vi "Begin.vi"(11 "Image Size":T1=enum."160x120") -> (0 "error out":errorcluster)   [LabVIEW 2012]
doc: "Called before other user functions, this VI is expected to open initial I/O refnums, load in file data, and do all program initialization. Notice that the <B>error out</B> terminal is simply used for data flow. Wiring it to other structures or subVIs ensures that this VI runs first."
uses:
  <vilib>/Rock Robotics/WPI/Camera/WPI_CameraImageSize.ctl
  <vilib>/Rock Robotics/WPI/Camera/WPI_CameraWhite Balance Values.ctl
  <vilib>/Rock Robotics/WPI/Camera/WPI_CameraExposure Values.ctl
  <vilib>/Rock Robotics/WPI/Camera/WPI_CameraFrameRate.ctl
  <vilib>/Rock Robotics/WPI/DriverStation/WPI_DriverStationRobotMode2.ctl
  <vilib>/Rock Robotics/WPI/Joystick/WPI_JoystickDeviceEnum.ctl
  <vilib>/Rock Robotics/SystemInterfaces/DIO/FPGA_DIOPWMChannel.ctl
  <vilib>/Rock Robotics/WPI/Solenoid/WPI_SolenoidChannel.ctl
  <vilib>/Rock Robotics/SystemInterfaces/DIO/FPGA_DIORelayChannel.ctl
  <vilib>/Rock Robotics/WPI/Relay/WPI_RelayDirection.ctl
  <vilib>/Rock Robotics/SystemInterfaces/DIO/FPGA_DIOChannel.ctl
  <vilib>/Rock Robotics/WPI/Encoder/WPI_EncoderType.ctl
  <vilib>/Rock Robotics/SystemInterfaces/Typedef/FPGA_TypedefDigitalModule.ctl
  <vilib>/Rock Robotics/SystemInterfaces/Typedef/FPGA_TypedefAnalogModuleForGyro.ctl
  <vilib>/Rock Robotics/SystemInterfaces/AI/FPGA_AIGyroChannel.ctl
  <vilib>/Rock Robotics/SystemInterfaces/Typedef/FPGA_TypedefSolenoidModule.ctl
  Robot Global Data.vi
  <vilib>/Rock Robotics/WPI/RobotDrive/WPI_RobotDriveOpen4MotorWithTalon.vi
  <vilib>/Rock Robotics/WPI/MotorControl/WPI_MotorControlOpen Talon.vi
  <vilib>/Rock Robotics/WPI/Solenoid/WPI_SolenoidOpenSingle.vi
  <vilib>/Rock Robotics/WPI/Solenoid/Deprecated/WPI_SolenoidSetBool.vi
  <vilib>/Rock Robotics/WPI/Counter/WPI_CounterDigitalInputToDigitalSource.vi
  <vilib>/Rock Robotics/WPI/MotorControl/WPI_MotorControlOpen Jaguar.vi
  <vilib>/Rock Robotics/WPI/Compressor/WPI_CompressorGetSetRefNum.vi
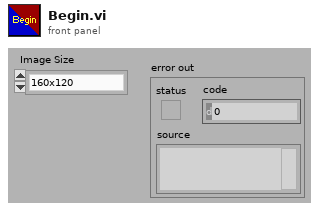
[diagram p1: front panel]
types:
  T1 = typedef "WPI_CameraImageSize.ctl" = enum16{"640x480", "320x240", "160x120"}
  T2 = typedef "FPGA_TypedefSolenoidModule.ctl" = enum16{"Solenoid Module 1", "Solenoid Module 2"}
  T3 = typedef "WPI_SolenoidChannel.ctl" = enum8{"Solenoid 1", "Solenoid 2", "Solenoid 3", "Solenoid 4", "Solenoid 5", "Solenoid 6", "Solenoid 7", "Solenoid 8", "Invalid"}
  T4 = typedef "FPGA_DIOPWMChannel.ctl" = enum8{"PWM 1", "PWM 2", "PWM 3", "PWM 4", "PWM 5", "PWM 6", "PWM 7", "PWM 8", "PWM 9", "PWM 10", "Invalid"}
  T5 = typedef "FPGA_TypedefDigitalModule.ctl" = enum16{"Digital Module 1", "Digital Module 2"}
  T6 = typedef "FPGA_AIGyroChannel.ctl" = enum8{"AI 1", "AI 2", "Invalid"}
  T7 = typedef "FPGA_TypedefAnalogModuleForGyro.ctl" = enum16{"Analog Module 1"}
  T8 = typedef "WPI_EncoderType.ctl" = enum16{"1x", "2x", "4x"}
  T9 = typedef "FPGA_DIOChannel.ctl" = enum8{"DIO 1", "DIO 2", "DIO 3", "DIO 4", "DIO 5", "DIO 6", "DIO 7", "DIO 8", "DIO 9", "DIO 10", "DIO 11", "DIO 12", "DIO 13", "DIO 14", "Invalid"}
  T10 = typedef "FPGA_DIORelayChannel.ctl" = enum8{"Relay 1", "Relay 2", "Relay 3", "Relay 4", "Relay 5", "Relay 6", "Relay 7", "Relay 8", "Invalid"}
  T11 = typedef "WPI_JoystickDeviceEnum.ctl" = enum16{"USB 1", "USB 2", "USB 3", "USB 4", "Kinect 1", "Kinect 2"}
  T12 = typedef "WPI_RelayDirection.ctl" = enum16{"Both directions", "Forward only", "Reverse only"}
  T13 = typedef "WPI_DriverStationRobotMode2.ctl" = enum16{"Autonomous Disabled", "Autonomous Enabled", "Teleop Disabled", "Teleop Enabled", "Timeout", "Finish", "Test Disabled", "Test Enabled"}
  T14 = typedef "WPI_CameraFrameRate.ctl" = u32
  T15 = typedef "WPI_CameraExposure Values.ctl" = enum16{"Auto", "Flicker-free 50 Hz", "Flicker-free 60 Hz", "Hold current"}
  T16 = typedef "WPI_CameraWhite Balance Values.ctl" = enum16{"Auto", "Fixed indoor", "Fixed outdoor 1", "Fixed outdoor 2", "Fixed fluorescent 1", "Fixed fluorescent 2", "Hold current"}
  T17 = typedef "WPI_MotorControlDeviceRef.ctl" = cluster{"DeviceStatus":errorcluster, "Type":enum16{"PWM", "CAN"}, "PWM":cluster{"Digital Module":T5, "PWM Channel":T4, "DeadBand":T18}, "CAN":cluster{"Device Number":u8, "Control Mode":T19, "Semaphore":T20, "Max Vout":dbl}, "Invert":bool, "TransformRef":T21, "InvTransformRef":T21}
  T18 = typedef "WPI_PWMDeadband.ctl" = cluster{"Name":string, "maxPositivePwm":i32, "minPositivePwm":i32, "centerPwm":i32, "maxNegativePwm":i32, "minNegativePwm":i32, "angularRange":u16}
  T19 = typedef "WPI_CANJaguar_ControlMode.ctl" = enum8{"Percent VBus", "Current", "Speed", "Position", "Voltage"}
  T20 = typedef "Semaphore RefNum" = refnum<k1>
  T21 = typedef "WPI_PWMTransform_ConPane.ctl" = refnum<vi>
  T22 = typedef "WPI_DigitalInputDevRef.ctl" = cluster{"DevStatus":errorcluster, "DIO Channel":T9, "Digital Module":T5}
  T23 = typedef "WPI_ServoDeviceRef.ctl" = cluster{"DeviceStatus":errorcluster, "Digital Module":T5, "PWM Channel":T4, "DeadBand":T18}
  T24 = typedef "WPI_JoystickDevRef.ctl" = cluster{"Device":T11}
  T25 = typedef "WPI_GyroDevRef.ctl" = cluster{"DevStatus":errorcluster, "Analog Module":T26, "Analog Channel":T27, "Offset":dbl, "Gain (VoltsPerDegree/Second)":dbl}
  T26 = typedef "FPGA_TypedefAnalogModule.ctl" = enum16{"Analog Module 1", "Analog Module 2"}
  T27 = typedef "FPGA_AIChannel.ctl" = enum8{"AI 1", "AI 2", "AI 3", "AI 4", "AI 5", "AI 6", "AI 7", "AI 8", "Invalid"}
  T28 = typedef "FPGA_CounterEncoderSourceConvertionLVSourceType.ctl" = cluster{"DevStatus":errorcluster, "AnalogTriggerMode?":bool, "DigitalMode":cluster{"Digital Module":T5, "DIO Channel":T29}, "AnalogTriggerMode":cluster{"AnalogTriggerIndex":T30, "OutputType":T31}}
  T29 = typedef "FPGA_DIODigitalSourceChannel.ctl" = enum8{"DIO 1", "DIO 2", "DIO 3", "DIO 4", "DIO 5", "DIO 6", "DIO 7", "DIO 8", "DIO 9", "DIO 10", "DIO 11", "DIO 12", "DIO 13", "DIO 14", "Disabled"}
  T30 = typedef "FPGA_AnalogTriggerIndex.ctl" = enum8{"Trig 0", "Trig 1", "Trig 2", "Trig 3", "Trig 4", "Trig 5", "Trig 6", "Trig 7", "Invalid"}
  T31 = typedef "FPGA_AnalogTriggerOutType.ctl" = enum16{"InWindow", "TriggerState", "Rising", "Falling"}
  T32 = typedef "WPI_SolenoidDevRef.ctl" = cluster{"DevStatus":errorcluster, "Solenoid Module":T2, "Forward Solenoid Channel":T3, "Reverse Solenoid Channel":T3}
  T33 = typedef "WPI_CompressorDevRef.ctl" = cluster{"DevStatus":errorcluster, "DigitalInputDevRef":T22, "RelayDevRef":T34}
  T34 = typedef "WPI_RelayDevRef.ctl" = cluster{"DevStatus":errorcluster, "Relay Channel":T10, "Digital Module":T5, "Relay Direction":T12}
  T35 = typedef "WPI_RobotDriveDevRef.ctl" = cluster{"DevStatus":errorcluster, "Motors[]":T17[], "Square Inputs":bool, "Max Output":dbl, "Isochronous":bool}
  T36 = typedef "WPI_EncoderDevRef.ctl" = cluster{"DevStatus":errorcluster, "EncoderIndex":T37, "CounterIndex":T38, "DistancePerCount":dbl, "Decoding Type":T8}
  T37 = typedef "FPGA_EncoderIdx.ctl" = enum8{"Enc 0", "Enc 1", "Enc 2", "Enc 3", "Invalid"}
  T38 = typedef "FPGA_CounterCtrSystemIndex.ctl" = enum8{"Ctr 0", "Ctr 1", "Ctr 2", "Ctr 3", "Ctr 4", "Ctr 5", "Ctr 6", "Ctr 7", "Invalid"}
  T39 = typedef "WPI_CameraDevRef.ctl" = cluster{"Camera Address":string, "CameraStatus":errorcluster, "Acquire Image Notifier":refnum<notifier>}
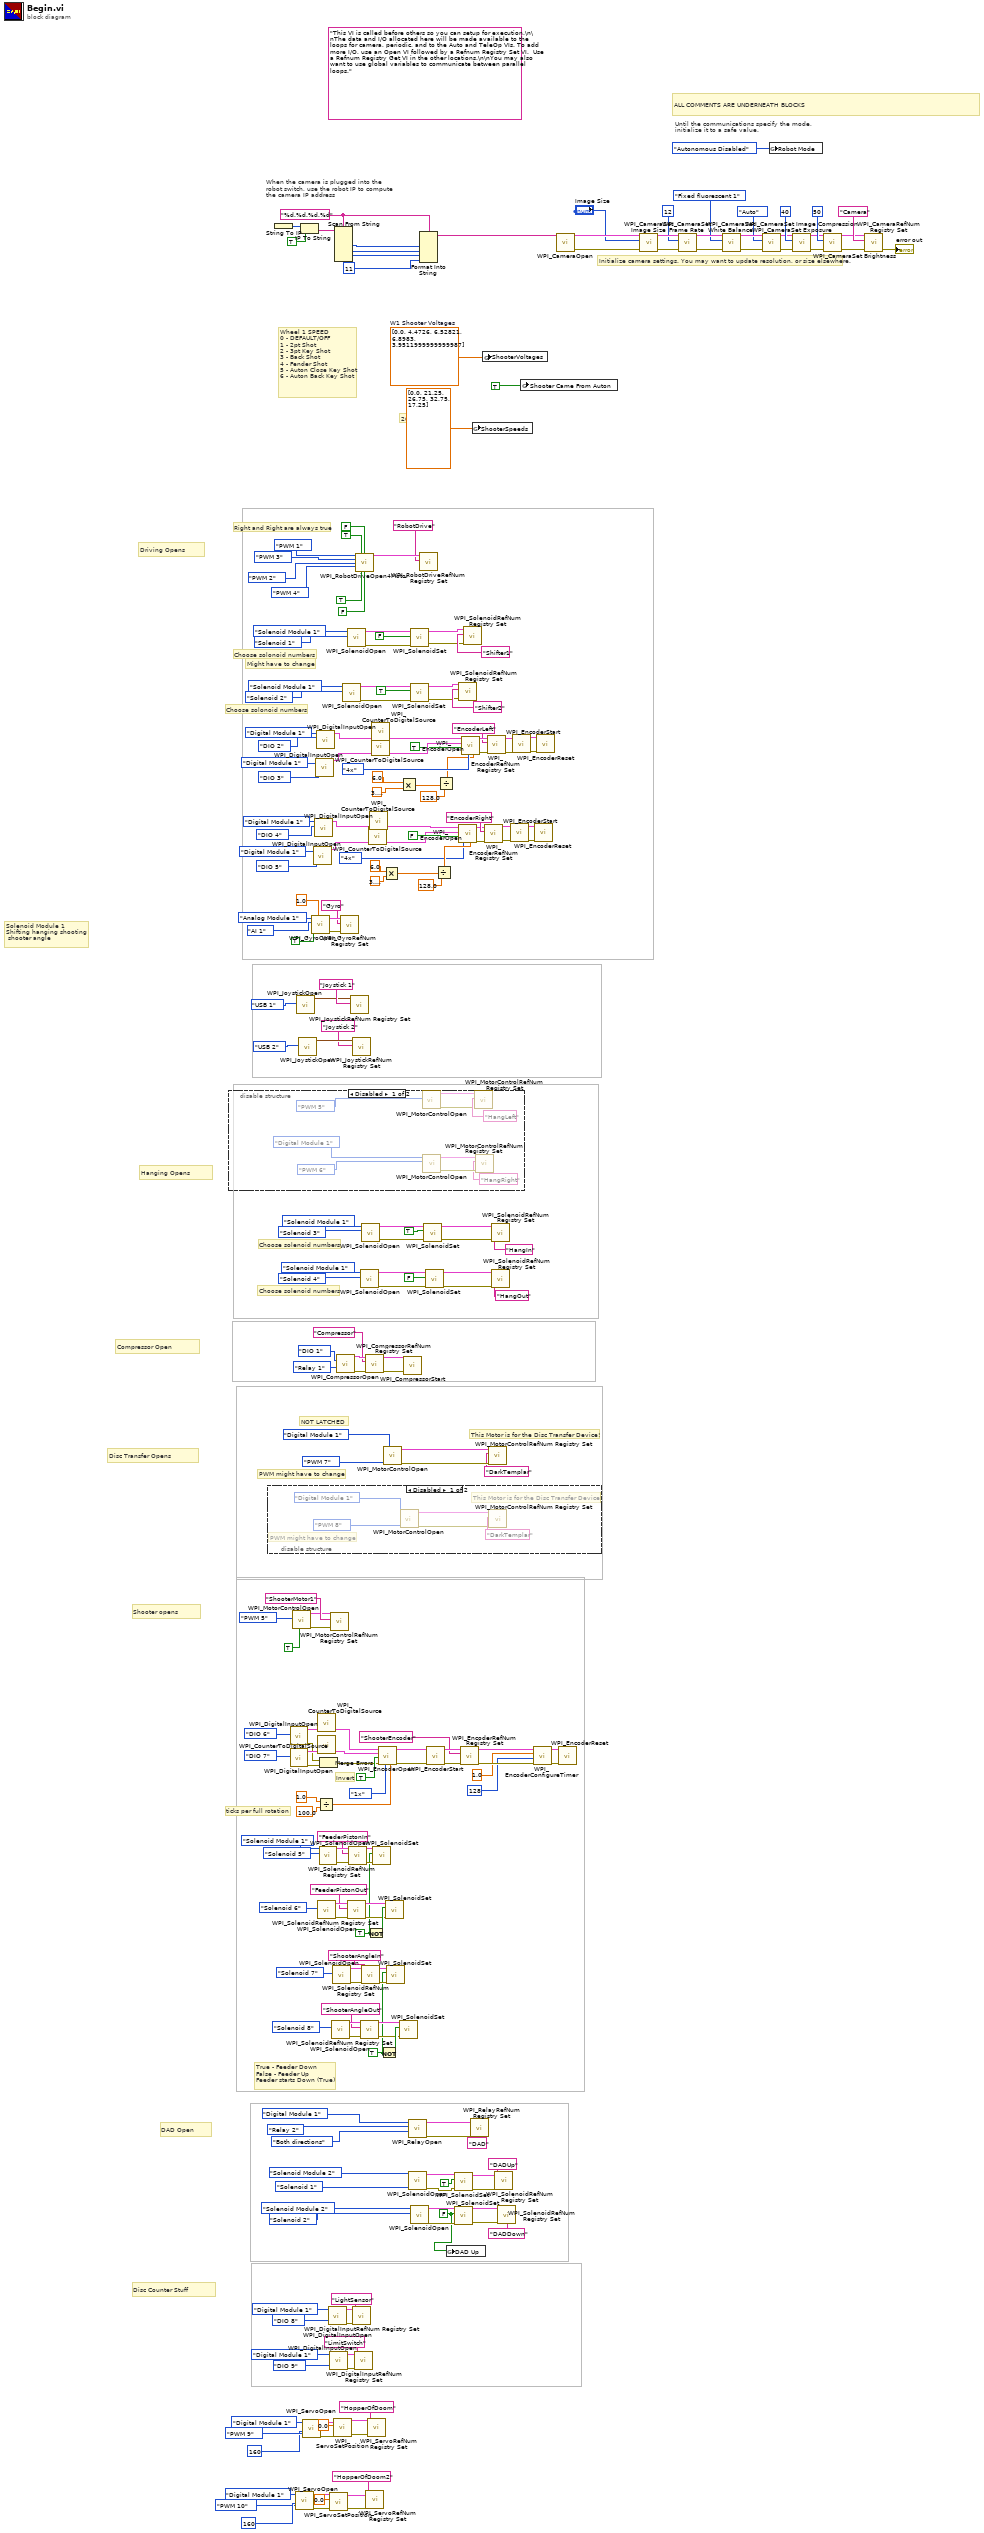
[diagram p0: block diagram]
diagram:
  w2 = TRUE
  w16 = TRUE
  w50 = FALSE
  w150 = dbl[] [0.0, 4.4726, 6.52821, 6.8983, 3.9511999999999987]  # W1 Shooter Voltages
  w227 = "%d.%d.%d.%d" ("format string")
  (unwired) "This VI is called before others so you can setup for execution.\n\nThe data and I/O allocated here will be made available to the loops for camera, periodic, and to the Auto and TeleOp VIs. To add more I/O, use an Open VI followed by a Refnum Registry Set VI.  Use a Refnum Registry Get VI in the other locations.\n\nYou may also want to use global variables to communicate between parallel loops."
  # "Solenoid Module 1\nShifting hanging shooting \n shooter angle"
  # "True - Feeder Down\nFalse - Feeder Up\nFeeder starts Down (True)"
  # "NOT LATCHED"
  # "Choose solenoid numbers"
  # "Choose solenoid numbers"
  # "Disc Counter Stuff"
  # "Compressor Open"
  # "26.75"
  # "Wheel 1 SPEED\n0 - DEFAULT/OFF\n1 - 2pt Shot\n2 - 3pt Key Shot\n3 - Back Shot\n4 - Fender Shot\n5 - Auton Close Key Shot\n6 - Auton Back Key Shot"
  # "Disc Transfer Opens"
  # "DAD Open"
  # "Hanging Opens"
  # "Driving Opens"
  # "Shooter opens"
  # "Invert"
  # "ticks per full rotation"
  # "Choose solonoid numbers"
  # "Might have to change"
  # "Choose solonoid numbers"
  # "PWM might have to change"
  # "ALL COMMENTS ARE UNDERNEATH BLOCKS"
  # "This Motor is for the Disc Transfer Device!"
  # "Right and Right are always true"
  # "Until the communications specify the mode,\ninitialize it to a safe value."
  # "When the camera is plugged into the\nrobot switch, use the robot IP to compute\nthe camera IP address"
  # "Initialize camera settings. You may want to update resolution, or size elsewhere."
  n1 = disable-structure shown="Disabled" {
    frame Disabled {
      n2 = call-poly <vilib>:"WPI_MotorControlOpen.vi"("PWM Channel"=FPGA_DIOPWMChannel."PWM 5") -> ("error out"=w258:errorcluster, "MotorControlDeviceRef"=w257:T17)  [unwired: 9 in]
      n3 = call-poly <vilib>:"WPI_MotorControlOpen.vi"("PWM Channel"=FPGA_DIOPWMChannel."PWM 6", "Digital Module (Module 1)"=FPGA_TypedefDigitalModule."Digital Module 1") -> ("error out"=w261:errorcluster, "MotorControlDeviceRef"=w262:T17)  [unwired: 8 in]
      n4 = call <vilib>:"WPI_MotorControlRefNum Registry Set.vi"("error in (no error)"=w258, "refnum name"="HangLeft", "MotorControlDevRef"=w257) -> ()  [unwired: 7 in, 2 out]
      n5 = call <vilib>:"WPI_MotorControlRefNum Registry Set.vi"("error in (no error)"=w261, "refnum name"="HangRight", "MotorControlDevRef"=w262) -> ()  [unwired: 7 in, 2 out]
    }
    frame Enabled {
    }
  }
  n6 = disable-structure shown="Disabled" {
    frame Disabled {
      # "PWM might have to change"
      # "This Motor is for the Disc Transfer Device!"
      n7 = call-poly <vilib>:"WPI_MotorControlOpen.vi"("PWM Channel"=FPGA_DIOPWMChannel."PWM 8", "Digital Module (Module 1)"=FPGA_TypedefDigitalModule."Digital Module 1") -> ("error out"=w268:errorcluster, "MotorControlDeviceRef"=w267:T17)  [unwired: 8 in]
      n8 = call <vilib>:"WPI_MotorControlRefNum Registry Set.vi"("error in (no error)"=w268, "refnum name"="DarkTemplar", "MotorControlDevRef"=w267) -> ()  [unwired: 7 in, 2 out]
    }
    frame Enabled {
    }
  }
  n9 = String To IP() -> (0:w234:u32)  [unwired: 1 in]
  n10 = call <vilib>:"WPI_DigitalInputOpen.vi"("DIO Channel"=FPGA_DIOChannel."DIO 6") -> ("error out"=w169:errorcluster, "DigitalInputDevRef"=w183:T22)  [unwired: 9 in]
  n11 = call <vilib>:"WPI_DigitalInputOpen.vi"("DIO Channel"=FPGA_DIOChannel."DIO 7") -> ("error out"=w168:errorcluster, "DigitalInputDevRef"=w179:T22)  [unwired: 9 in]
  n12 = call-poly <vilib>:"WPI_MotorControlOpen.vi"("Invert"=TRUE, "PWM Channel"=FPGA_DIOPWMChannel."PWM 5") -> ("error out"=w162:errorcluster, "MotorControlDeviceRef"=w163:T17)  [unwired: 8 in]
  n13 = call <vilib>:"WPI_ServoOpen.vi"("Angular Range"=160, "PWM Channel"=FPGA_DIOPWMChannel."PWM 10", "Digital Module (Module 1)"=FPGA_TypedefDigitalModule."Digital Module 1") -> ("error out"=w35:errorcluster, "ServoDeviceRef"=w34:T23)  [unwired: 7 in]
  n14 = call <vilib>:"WPI_JoystickOpen.vi"("JoystickDevice"=WPI_JoystickDeviceEnum."USB 1") -> ("JoystickDevRef"=w223:T24)  [unwired: 10 in]
  n15 = call <vilib>:"WPI_JoystickOpen.vi"("JoystickDevice"=WPI_JoystickDeviceEnum."USB 2") -> ("JoystickDevRef"=w152:T24)  [unwired: 10 in]
  n16 = IP To String(1:TRUE ("dot notation? (F)"), 2:w234) -> (0:w232:string)
  n17 = call <vilib>:"WPI_ServoOpen.vi"("Angular Range"=160, "PWM Channel"=FPGA_DIOPWMChannel."PWM 9", "Digital Module (Module 1)"=FPGA_TypedefDigitalModule."Digital Module 1") -> ("error out"=w39:errorcluster, "ServoDeviceRef"=w38:T23)  [unwired: 7 in]
  n18 = call <vilib>:"WPI_GyroOpen.vi"("Calibration Time (s)"=1.0, "Calibrate On Open"=TRUE, "Analog Channel"=FPGA_AIGyroChannel."AI 1", "Analog Module (Module 1)"=FPGA_TypedefAnalogModuleForGyro."Analog Module 1") -> ("error out"=w88:errorcluster, "GyroDevRef"=w87:T25)  [unwired: 5 in, 1 out]
  n19 = call <vilib>:"WPI_DigitalInputOpen.vi"("DIO Channel"=FPGA_DIOChannel."DIO 5", "Digital Module (Module 1)"=FPGA_TypedefDigitalModule."Digital Module 1") -> ("DigitalInputDevRef"=w96:T22)  [unwired: 8 in, 1 out]
  n20 = call <vilib>:"WPI_DigitalInputOpen.vi"("DIO Channel"=FPGA_DIOChannel."DIO 4", "Digital Module (Module 1)"=FPGA_TypedefDigitalModule."Digital Module 1") -> ("DigitalInputDevRef"=w95:T22)  [unwired: 8 in, 1 out]
  n21 = call <vilib>:"WPI_DigitalInputOpen.vi"("DIO Channel"=FPGA_DIOChannel."DIO 3", "Digital Module (Module 1)"=FPGA_TypedefDigitalModule."Digital Module 1") -> ("DigitalInputDevRef"=w125:T22)  [unwired: 8 in, 1 out]
  n22 = call <vilib>:"WPI_DigitalInputOpen.vi"("DIO Channel"=FPGA_DIOChannel."DIO 2", "Digital Module (Module 1)"=FPGA_TypedefDigitalModule."Digital Module 1") -> ("DigitalInputDevRef"=w126:T22)  [unwired: 8 in, 1 out]
  n23 = Divide(x=1.0, y=100.0) -> (x/y=w157:dbl)
  n24 = call-poly <vilib>:"WPI_CounterToDigitalSource.vi"("DigitalInputDevRef"=w183) -> ("Digital Source"=w182:T28)  [unwired: 6 in]
  n25 = call-poly <vilib>:"WPI_CounterToDigitalSource.vi"("DigitalInputDevRef"=w179) -> ("Digital Source"=w176:T28)  [unwired: 6 in]
  n26 = call-poly <vilib>:"WPI_SolenoidOpen.vi"("Solenoid Channel"=WPI_SolenoidChannel."Solenoid 6") -> ("error out"=w26:errorcluster, "SolenoidDevRef"=w25:T32)  [unwired: 9 in]
  n27 = call-poly <vilib>:"WPI_SolenoidOpen.vi"("Solenoid Channel"=WPI_SolenoidChannel."Solenoid 5", "Solenoid Module (Module 1)"=FPGA_TypedefSolenoidModule."Solenoid Module 1") -> ("error out"=w21:errorcluster, "SolenoidDevRef"=w22:T32)  [unwired: 8 in]
  n28 = Merge Errors(w169, w168) -> (w170:errorcluster)
  n29 = call <vilib>:"WPI_DigitalInputOpen.vi"("DIO Channel"=FPGA_DIOChannel."DIO 8", "Digital Module (Module 1)"=FPGA_TypedefDigitalModule."Digital Module 1") -> ("error out"=w142:errorcluster, "DigitalInputDevRef"=w141:T22)  [unwired: 8 in]
  n30 = call <vilib>:"WPI_DigitalInputOpen.vi"("DIO Channel"=FPGA_DIOChannel."DIO 9", "Digital Module (Module 1)"=FPGA_TypedefDigitalModule."Digital Module 1") -> ("error out"=w140:errorcluster, "DigitalInputDevRef"=w139:T22)  [unwired: 8 in]
  n31 = call <vilib>:"WPI_ServoSetPosition.vi"("error in (no error)"=w35, "Position"=0.0, "ServoDeviceRef"=w34) -> ("error out"=w32:errorcluster, "ServoDeviceRef"=w33:T23)  [unwired: 7 in]
  n32 = call <vilib>:"WPI_MotorControlRefNum Registry Set.vi"("error in (no error)"=w162, "refnum name"="ShooterMotor1", "MotorControlDevRef"=w163) -> ()  [unwired: 7 in, 2 out]
  n33 = call-poly <vilib>:"WPI_SolenoidOpen.vi"("Solenoid Channel"=WPI_SolenoidChannel."Solenoid 8") -> ("error out"=w12:errorcluster, "SolenoidDevRef"=w11:T32)  [unwired: 9 in]
  n34 = call-poly <vilib>:"WPI_SolenoidOpen.vi"("Solenoid Channel"=WPI_SolenoidChannel."Solenoid 7") -> ("error out"=w7:errorcluster, "SolenoidDevRef"=w8:T32)  [unwired: 9 in]
  n35 = call <vilib>:"WPI_ServoSetPosition.vi"("error in (no error)"=w39, "Position"=0.0, "ServoDeviceRef"=w38) -> ("error out"=w37:errorcluster, "ServoDeviceRef"=w36:T23)  [unwired: 7 in]
  n36 = Scan From String(format string=w227, input string=w232) -> (output 1=w231:i32, output 2=w230:i32, output 3=w229:i32)  [unwired: 7 in, 3 out]
  n37 = call <vilib>:"WPI_CompressorOpen.vi"("Pressure Switch DIO Channel"=FPGA_DIOChannel."DIO 1", "Relay Channel"=FPGA_DIORelayChannel."Relay 1") -> ("CompressorDevRef"=w148:T33, "error out"=w146:errorcluster)  [unwired: 12 in]
  n38 = call <vilib>:"WPI_GyroRefNum Registry Set.vi"("error in (no error)"=w88, "refnum name"="Gyro", "GyroDevRef"=w87) -> ()  [unwired: 7 in, 2 out]
  n39 = call-poly <vilib>:"WPI_SolenoidOpen.vi"("Solenoid Channel"=WPI_SolenoidChannel."Solenoid 2", "Solenoid Module (Module 1)"=FPGA_TypedefSolenoidModule."Solenoid Module 1") -> ("error out"=w191:errorcluster, "SolenoidDevRef"=w193:T32)  [unwired: 8 in]
  n40 = call-poly <vilib>:"WPI_SolenoidOpen.vi"("Solenoid Channel"=WPI_SolenoidChannel."Solenoid 1", "Solenoid Module (Module 1)"=FPGA_TypedefSolenoidModule."Solenoid Module 1") -> ("error out"=w196:errorcluster, "SolenoidDevRef"=w199:T32)  [unwired: 8 in]
  n41 = call <vilib>:"WPI_SolenoidRefNum Registry Set.vi"("error in (no error)"=w26, "refnum name"="FeederPistonOut", "SolenoidDevRef"=w25) -> ("error out"=w28:errorcluster, "SolenoidDevRef"=w27:T32)  [unwired: 7 in]
  n42 = call <vilib>:"WPI_SolenoidRefNum Registry Set.vi"("error in (no error)"=w21, "refnum name"="FeederPistonIn", "SolenoidDevRef"=w22) -> ("error out"=w19:errorcluster, "SolenoidDevRef"=w20:T32)  [unwired: 7 in]
  n43 = call <vilib>:"WPI_JoystickRefNum Registry Set.vi"("refnum name"="Joystick 1", "JoystickDevRef"=w223) -> ()  [unwired: 8 in, 2 out]
  n44 = call <vilib>:"WPI_JoystickRefNum Registry Set.vi"("refnum name"="Joystick 2", "JoystickDevRef"=w152) -> ()  [unwired: 8 in, 2 out]
  n45 = call <vilib>:"WPI_DigitalInputRefNum Registry Set.vi"("error in (no error)"=w142, "refnum name"="LightSensor", "DigitalInputDevRef"=w141) -> ()  [unwired: 7 in, 2 out]
  n46 = call <vilib>:"WPI_DigitalInputRefNum Registry Set.vi"("error in (no error)"=w140, "refnum name"="LimitSwitch", "DigitalInputDevRef"=w139) -> ()  [unwired: 7 in, 2 out]
  n47 = call-poly <vilib>:"WPI_RobotDriveOpen4Motor.vi"("Rear Left Motor"=FPGA_DIOPWMChannel."PWM 1", "Rear Left Motor Inverted"=TRUE, "Rear Right Motor Inverted"=FALSE, "Rear Right Motor"=FPGA_DIOPWMChannel."PWM 3", "Front Left Motor"=FPGA_DIOPWMChannel."PWM 2", "Front Right Motor"=FPGA_DIOPWMChannel."PWM 4" ("Front Left Motor"), "Front Left Motor Inverted"=TRUE, "Front Right Motor Inverted"=FALSE) -> ("RobotDriveDevRef"=w212:T35)  [unwired: 6 in, 1 out]
  n48 = call-poly <vilib>:"WPI_SolenoidOpen.vi"("Solenoid Channel"=WPI_SolenoidChannel."Solenoid 4", "Solenoid Module (Module 1)"=FPGA_TypedefSolenoidModule."Solenoid Module 1") -> ("error out"=w72:errorcluster, "SolenoidDevRef"=w73:T32)  [unwired: 8 in]
  n49 = call <vilib>:"WPI_SolenoidRefNum Registry Set.vi"("error in (no error)"=w12, "refnum name"="ShooterAngleOut", "SolenoidDevRef"=w11) -> ("error out"=w14:errorcluster, "SolenoidDevRef"=w13:T32)  [unwired: 7 in]
  n50 = call-poly <vilib>:"WPI_SolenoidOpen.vi"("Solenoid Channel"=WPI_SolenoidChannel."Solenoid 3", "Solenoid Module (Module 1)"=FPGA_TypedefSolenoidModule."Solenoid Module 1") -> ("error out"=w75:errorcluster, "SolenoidDevRef"=w74:T32)  [unwired: 8 in]
  n51 = call <vilib>:"WPI_SolenoidRefNum Registry Set.vi"("error in (no error)"=w7, "refnum name"="ShooterAngleIn", "SolenoidDevRef"=w8) -> ("error out"=w5:errorcluster, "SolenoidDevRef"=w6:T32)  [unwired: 7 in]
  n52 = call <vilib>:"WPI_CompressorRefNum Registry Set.vi"("error in (no error)"=w146, "refnum name"="Compressor", "CompressorDevRef"=w148) -> ("error out"=w48:errorcluster, "CompressorDevRef"=w49:T33)  [unwired: 7 in]
  n53 = call <vilib>:"WPI_ServoRefNum Registry Set.vi"("error in (no error)"=w32, "refnum name"="HopperOfDoom2", "ServoDeviceRef"=w33) -> ()  [unwired: 7 in, 2 out]
  n54 = Not(x=w16) -> (.not. x?=w29:bool)
  n55 = call <vilib>:"WPI_ServoRefNum Registry Set.vi"("error in (no error)"=w37, "refnum name"="HopperOfDoom", "ServoDeviceRef"=w36) -> ()  [unwired: 7 in, 2 out]
  n56 = call-poly <vilib>:"WPI_CounterToDigitalSource.vi"("DigitalInputDevRef"=w96) -> ("Digital Source"=w92:T28)  [unwired: 6 in]
  n57 = call-poly <vilib>:"WPI_CounterToDigitalSource.vi"("DigitalInputDevRef"=w95) -> ("Digital Source"=w90:T28)  [unwired: 6 in]
  n58 = call-poly <vilib>:"WPI_CounterToDigitalSource.vi"("DigitalInputDevRef"=w125) -> ("Digital Source"=w129:T28)  [unwired: 6 in]
  n59 = call-poly <vilib>:"WPI_CounterToDigitalSource.vi"("DigitalInputDevRef"=w126) -> ("Digital Source"=w132:T28)  [unwired: 6 in]
  n60 = call-poly <vilib>:"WPI_SolenoidSet.vi"("error in (no error)"=w19, "Value"=w16, "SolenoidDevRef"=w20) -> ()  [unwired: 7 in, 2 out]
  n61 = call <vilib>:"WPI_EncoderOpen.vi"("DistancePerCount"=w157, "Decoding Type"=WPI_EncoderType."1x", "error in (no error)"=w170, "Invert Direction (False)"=TRUE, "BSource"=w176, "ASource"=w182) -> ("error out"=w171:errorcluster, "EncoderDevRef"=w172:T36)  [unwired: 4 in]
  n62 = Not(x=w2) -> (.not. x?=w15:bool)
  n63 = Multiply(x=6.0, y=3.141592653589793) -> (x*y=w101:dbl)
  n64 = call-poly <vilib>:"WPI_MotorControlOpen.vi"("PWM Channel"=FPGA_DIOPWMChannel."PWM 7", "Digital Module (Module 1)"=FPGA_TypedefDigitalModule."Digital Module 1") -> ("error out"=w207:errorcluster, "MotorControlDeviceRef"=w208:T17)  [unwired: 8 in]
  n65 = call-poly <vilib>:"WPI_SolenoidSet.vi"("error in (no error)"=w28, "Value"=w29, "SolenoidDevRef"=w27) -> ()  [unwired: 7 in, 2 out]
  n66 = call-poly <vilib>:"WPI_SolenoidSet.vi"("error in (no error)"=w5, "Value"=w2, "SolenoidDevRef"=w6) -> ()  [unwired: 7 in, 2 out]
  n67 = call-poly <vilib>:"WPI_SolenoidSet.vi"("error in (no error)"=w14, "Value"=w15, "SolenoidDevRef"=w13) -> ()  [unwired: 7 in, 2 out]
  n68 = Multiply(x=6.0, y=3.141592653589793) -> (x*y=w120:dbl)
  n69 = call <vilib>:"WPI_CompressorStart.vi"("error in (no error)"=w48, "CompressorDevRef"=w49) -> ()  [unwired: 8 in, 2 out]
  n70 = call <vilib>:"WPI_RelayOpen.vi"("Relay Direction"=WPI_RelayDirection."Both directions", "Relay Channel"=FPGA_DIORelayChannel."Relay 2", "Digital Module (Module 1)"=FPGA_TypedefDigitalModule."Digital Module 1") -> ("error out"=w186:errorcluster, "RelayDevRef"=w185:T34)  [unwired: 7 in]
  n71 = call-poly <vilib>:"WPI_SolenoidOpen.vi"("Solenoid Channel"=WPI_SolenoidChannel."Solenoid 1", "Solenoid Module (Module 1)"=FPGA_TypedefSolenoidModule."Solenoid Module 2") -> ("error out"=w54:errorcluster, "SolenoidDevRef"=w59:T32)  [unwired: 8 in]
  n72 = call-poly <vilib>:"WPI_SolenoidSet.vi"("error in (no error)"=w191, "Value"=TRUE, "SolenoidDevRef"=w193) -> ("error out"=w190:errorcluster, "SolenoidDevRef"=w192:T32)  [unwired: 7 in]
  n73 = call-poly <vilib>:"WPI_SolenoidOpen.vi"("Solenoid Channel"=WPI_SolenoidChannel."Solenoid 2", "Solenoid Module (Module 1)"=FPGA_TypedefSolenoidModule."Solenoid Module 2") -> ("error out"=w51:errorcluster, "SolenoidDevRef"=w56:T32)  [unwired: 8 in]
  n74 = call-poly <vilib>:"WPI_SolenoidSet.vi"("error in (no error)"=w196, "Value"=FALSE, "SolenoidDevRef"=w199) -> ("error out"=w197:errorcluster, "SolenoidDevRef"=w198:T32)  [unwired: 7 in]
  n75 = Format Into String(format string=w227, w231, w230, w229, 11 ("Compression")) -> (resulting string=w225:string)  [unwired: 2 in, 1 out]
  n76 = call <vilib>:"WPI_RobotDriveRefNum Registry Set.vi"("refnum name"="RobotDrive", "RobotDriveDevRef"=w212) -> ()  [unwired: 8 in, 2 out]
  n77 = call-poly <vilib>:"WPI_SolenoidSet.vi"("error in (no error)"=w75, "Value"=TRUE, "SolenoidDevRef"=w74) -> ("error out"=w68:errorcluster, "SolenoidDevRef"=w71:T32)  [unwired: 7 in]
  n78 = call-poly <vilib>:"WPI_SolenoidSet.vi"("error in (no error)"=w72, "Value"=FALSE, "SolenoidDevRef"=w73) -> ("error out"=w69:errorcluster, "SolenoidDevRef"=w70:T32)  [unwired: 7 in]
  n79 = call <vilib>:"WPI_EncoderStart.vi"("error in (no error)"=w171, "EncoderDevRef"=w172) -> ("error out"=w167:errorcluster, "EncoderDevRef"=w173:T36)  [unwired: 8 in]
  n80 = Divide(x=w101, y=128.0 ("x")) -> (x/y=w102:dbl)
  n81 = Divide(x=w120, y=128.0 ("x")) -> (x/y=w119:dbl)
  n82 = global write "Robot Global Data.vi" "DAD Up"(w50) -> ()
  n83 = call-poly <vilib>:"WPI_SolenoidSet.vi"("error in (no error)"=w54, "Value"=TRUE, "SolenoidDevRef"=w59) -> ("error out"=w53:errorcluster, "SolenoidDevRef"=w57:T32)  [unwired: 7 in]
  n84 = call-poly <vilib>:"WPI_SolenoidSet.vi"("error in (no error)"=w51, "Value"=w50, "SolenoidDevRef"=w56) -> ("error out"=w52:errorcluster, "SolenoidDevRef"=w55:T32)  [unwired: 7 in]
  n85 = call <vilib>:"WPI_SolenoidRefNum Registry Set.vi"("error in (no error)"=w190, "refnum name"="Shifter2", "SolenoidDevRef"=w192) -> ()  [unwired: 7 in, 2 out]
  n86 = call <vilib>:"WPI_EncoderOpen.vi"("DistancePerCount"=w102, "Decoding Type"=WPI_EncoderType."4x", "Invert Direction (False)"=FALSE, "BSource"=w92, "ASource"=w90) -> ("error out"=w103:errorcluster, "EncoderDevRef"=w104:T36)  [unwired: 5 in]
  n87 = call <vilib>:"WPI_EncoderRefNum Registry Set.vi"("error in (no error)"=w167, "refnum name"="ShooterEncoder", "EncoderDevRef"=w173) -> ("error out"=w158:errorcluster, "EncoderDevRef"=w159:T36)  [unwired: 7 in]
  n88 = call <vilib>:"WPI_EncoderOpen.vi"("DistancePerCount"=w119, "Decoding Type"=WPI_EncoderType."4x", "Invert Direction (False)"=TRUE, "BSource"=w129, "ASource"=w132) -> ("error out"=w118:errorcluster, "EncoderDevRef"=w117:T36)  [unwired: 5 in]
  n89 = call <vilib>:"WPI_SolenoidRefNum Registry Set.vi"("error in (no error)"=w197, "refnum name"="Shifter1", "SolenoidDevRef"=w198) -> ()  [unwired: 7 in, 2 out]
  n90 = call <vilib>:"WPI_RelayRefNum Registry Set.vi"("error in (no error)"=w186, "refnum name"="DAD", "RelayDevRef"=w185) -> ()  [unwired: 7 in, 2 out]
  n91 = global write "Robot Global Data.vi" "ShooterSpeeds"(dbl[] [0.0, 21.25, 26.75, 32.75, 17.25]) -> ()
  n92 = global write "Robot Global Data.vi" "ShooterVoltages"(w150) -> ()
  n93 = call <vilib>:"WPI_EncoderRefNum Registry Set.vi"("error in (no error)"=w103, "refnum name"="EncoderRight", "EncoderDevRef"=w104) -> ("error out"=w106:errorcluster, "EncoderDevRef"=w107:T36)  [unwired: 7 in]
  n94 = call <vilib>:"WPI_EncoderRefNum Registry Set.vi"("error in (no error)"=w118, "refnum name"="EncoderLeft", "EncoderDevRef"=w117) -> ("error out"=w115:errorcluster, "EncoderDevRef"=w114:T36)  [unwired: 7 in]
  n95 = call <vilib>:"WPI_MotorControlRefNum Registry Set.vi"("error in (no error)"=w207, "refnum name"="DarkTemplar", "MotorControlDevRef"=w208) -> ()  [unwired: 7 in, 2 out]
  n96 = call <vilib>:"WPI_SolenoidRefNum Registry Set.vi"("error in (no error)"=w68, "refnum name"="HangIn", "SolenoidDevRef"=w71) -> ()  [unwired: 7 in, 2 out]
  n97 = call <vilib>:"WPI_SolenoidRefNum Registry Set.vi"("error in (no error)"=w69, "refnum name"="HangOut", "SolenoidDevRef"=w70) -> ()  [unwired: 7 in, 2 out]
  n98 = call <vilib>:"WPI_SolenoidRefNum Registry Set.vi"("error in (no error)"=w53, "refnum name"="DADUp", "SolenoidDevRef"=w57) -> ()  [unwired: 7 in, 2 out]
  n99 = call <vilib>:"WPI_SolenoidRefNum Registry Set.vi"("error in (no error)"=w52, "refnum name"="DADDown", "SolenoidDevRef"=w55) -> ()  [unwired: 7 in, 2 out]
  n100 = call <vilib>:"WPI_EncoderStart.vi"("error in (no error)"=w106, "EncoderDevRef"=w107) -> ("error out"=w108:errorcluster, "EncoderDevRef"=w109:T36)  [unwired: 8 in]
  n101 = call <vilib>:"WPI_EncoderStart.vi"("error in (no error)"=w115, "EncoderDevRef"=w114) -> ("error out"=w113:errorcluster, "EncoderDevRef"=w112:T36)  [unwired: 8 in]
  n102 = global write "Robot Global Data.vi" "Shooter Came From Auton"(TRUE) -> ()
  n103 = call <vilib>:"WPI_EncoderConfigureTimer.vi"("error in (no error)"=w158, "Number Samples to Average"=u8 128, "Minimum Rate"=1.0, "EncoderDevRef"=w159) -> ("error out"=w161:errorcluster, "EncoderDevRef"=w160:T36)  [unwired: 6 in]
  n104 = call <vilib>:"WPI_EncoderReset.vi"("error in (no error)"=w108, "EncoderDevRef"=w109) -> ()  [unwired: 8 in, 2 out]
  n105 = call <vilib>:"WPI_EncoderReset.vi"("error in (no error)"=w113, "EncoderDevRef"=w112) -> ()  [unwired: 8 in, 2 out]
  n106 = call <vilib>:"WPI_CameraOpen.vi"("Camera Address"=w225) -> ("error out"=w246:errorcluster, "CameraDevRef"=w247:T39)  [unwired: 1 in, 8 out]
  n107 = call <vilib>:"WPI_EncoderReset.vi"("error in (no error)"=w161, "EncoderDevRef"=w160) -> ()  [unwired: 8 in, 2 out]
  n108 = call <vilib>:"WPI_CameraSet Image Size.vi"("error in (no error)"=w246, "Image Size"="Image Size", "CameraDevRef"=w247) -> ("error out"=w245:errorcluster, "CameraDevRef Out"=w248:T39)  [unwired: 7 out]
  n109 = call <vilib>:"WPI_CameraSet Frame Rate.vi"("error in (no error)"=w245, "Frame Rate (fps)"=T14 12, "CameraDevRef"=w248) -> ("error out"=w244:errorcluster, "CameraDevRef Out"=w250:T39)  [unwired: 7 out]
  n110 = call <vilib>:"WPI_CameraSet White Balance.vi"("error in (no error)"=w244, "White Balance"=WPI_CameraWhite_Balance_Values."Fixed fluorescent 1", "CameraDevRef"=w250) -> ("error out"=w243:errorcluster, "CameraDevRef Out"=w249:T39)  [unwired: 7 out]
  n111 = call <vilib>:"WPI_CameraSet Exposure.vi"("error in (no error)"=w243, "Exposure"=WPI_CameraExposure_Values."Auto", "CameraDevRef"=w249) -> ("error out"=w242:errorcluster, "CameraDevRef Out"=w252:T39)  [unwired: 7 out]
  n112 = global write "Robot Global Data.vi" "Robot Mode"(WPI_DriverStationRobotMode2."Autonomous Disabled" ("Robot Mode")) -> ()
  n113 = call <vilib>:"WPI_CameraSet Image Compression.vi"("error in (no error)"=w242, "Compression"=40, "CameraDevRef"=w252) -> ("error out"=w241:errorcluster, "CameraDevRef Out"=w251:T39)  [unwired: 7 out]
  n114 = call <vilib>:"WPI_CameraSet Brightness.vi"("error in (no error)"=w241, "Brightness"=50, "CameraDevRef"=w251) -> ("error out"=w239:errorcluster, "CameraDevRef Out"=w240:T39)  [unwired: 7 out]
  n115 = call <vilib>:"WPI_CameraRefNum Registry Set.vi"("error in (no error)"=w239, "refnum name"="Camera", "CameraDevRef"=w240) -> ("error out"=→"error out":errorcluster)  [unwired: 8 out]
